vi "pubEventCpp_summaryState.vi"(8 "error in (no error)":errorcluster, 10 "pathOfSendEventSummaryState":path, 11 "SalProcess in":refnum<class "SalProcess.lvclass">) -> (0 "error out":errorcluster, 3 "SalProcess out":refnum<class "SalProcess.lvclass">)   [LabVIEW 2018, in "SalProcess.lvclass"]
doc: "Publish the event by CPP (summary state.)"
uses:
  SalProcess.lvclass
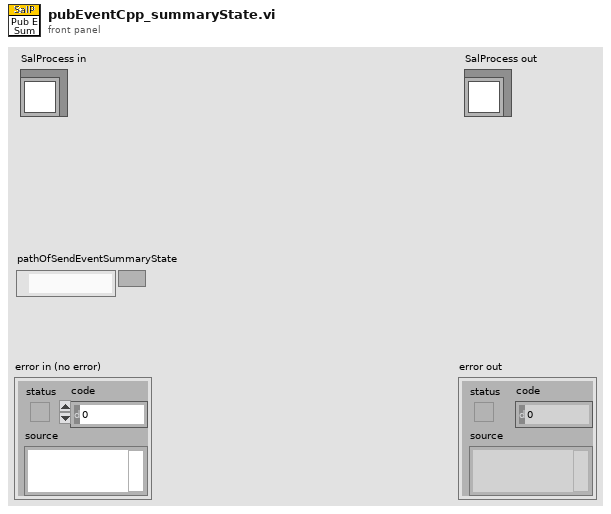
[diagram p1: front panel]
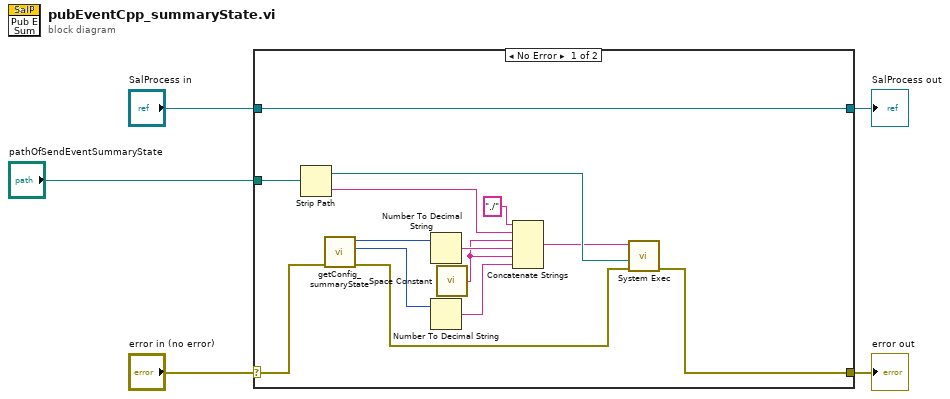
[diagram p0: block diagram]
diagram:
  n1 = case shown="No Error" "error in (no error)" {
    selector: "error in (no error)" -> [w18 w21]
    tunnel: [w12 w21] -> w4
    tunnel: [w19 w20] -> w2
    tunnel: "SalProcess in" -> [w19 w20]
    tunnel: "pathOfSendEventSummaryState" -> [w11 _]
    frame No Error {
      n2 = Strip Path(path=w11) -> (stripped path=w10:path, name=w9:string)
      n3 = call "getConfig_summaryState.vi"("error in (no error)"=w18) -> ("error out"=w13:errorcluster, "priority"=w16:i32, "summaryState"=w17:i32)  [unwired: 8 in]
      n4 = Number To Decimal String(number=w17) -> (decimal integer string=w15:string)  [unwired: 1 in]
      n5 = Number To Decimal String(number=w16) -> (decimal integer string=w14:string)  [unwired: 1 in]
      n6 = call <vilib>:"Space Constant.vi"() -> ("String"=w8:string)
      n7 = Concatenate Strings("./" ("string"), w9, w8, w15, w8, w14) -> (w6:string)
      n8 = call <vilib>:"System Exec.vi"("error in (no error)"=w13, "working directory"=w10, "command line"=w6) -> ("error out"=w12:errorcluster)  [unwired: 5 in, 3 out]
    }
    frame Error {
    }
  }
  "error out" <- w4
  "SalProcess out" <- w2
